vi "Index To Pair.vi"(11 "Index":i32) -> (2 "Second":u8, 3 "First":u8)   [LabVIEW 2020]
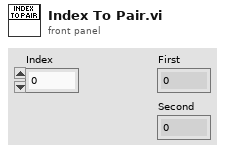
[diagram p1: front panel]
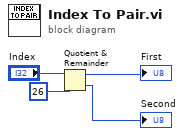
[diagram p0: block diagram]
diagram:
  n1 = Quotient & Remainder(x="Index", y=26) -> (x-y*floor(x/y)=→"First":i32, floor(x/y)=→"Second":i32)
